vi "RPT_Convert Waveform.vi"(11 "Wave Data IN":dbl[][](array[numeric])) -> (0 "appended array":dbl[][](array[numeric]), 2 "Text OUT":string[][](array[string]), 3 "Count":i32)   [LabVIEW 2024]
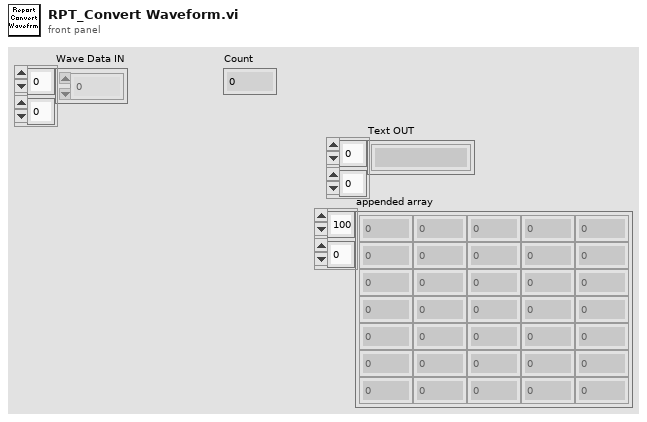
[diagram p1: front panel]
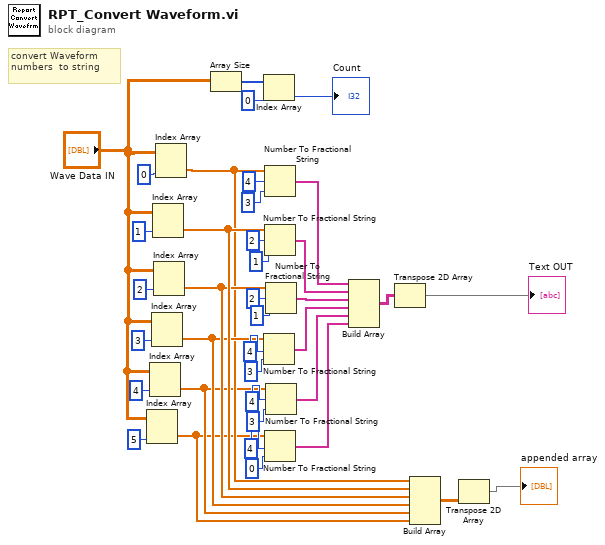
[diagram p0: block diagram]
diagram:
  # "convert Waveform\nnumbers  to string"
  n1 = Index Array(array="Wave Data IN", index (col)=5 ("index")) -> (element=w1:dbl[])  [unwired: 1 in]
  n2 = Index Array(array="Wave Data IN", index (col)=4 ("index")) -> (element=w2:dbl[])  [unwired: 1 in]
  n3 = Index Array(array="Wave Data IN", index (col)=3 ("index")) -> (element=w15:dbl[])  [unwired: 1 in]
  n4 = Index Array(array="Wave Data IN", index (col)=1 ("index")) -> (element=w17:dbl[])  [unwired: 1 in]
  n5 = Index Array(array="Wave Data IN", index (col)=2 ("index")) -> (element=w16:dbl[])  [unwired: 1 in]
  n6 = Index Array(array="Wave Data IN", index (col)=0 ("index")) -> (element=w12:dbl[])  [unwired: 1 in]
  n7 = Array Size(array="Wave Data IN") -> (size(s)=w26:i32[])
  n8 = Index Array(array=w26, index=0) -> (element=→"Count":i32)
  n9 = Number To Fractional String(number=w15, width (-)=i16 4 ("precision (6)"), precision (6)=i16 3) -> (F-format string=w36:string[])  [unwired: 1 in]
  n10 = Number To Fractional String(number=w12, width (-)=i16 4 ("precision (6)"), precision (6)=i16 3) -> (F-format string=w24:string[])  [unwired: 1 in]
  n11 = Number To Fractional String(number=w17, width (-)=i16 2 ("precision (6)"), precision (6)=i16 1) -> (F-format string=w30:string[])  [unwired: 1 in]
  n12 = Number To Fractional String(number=w1, width (-)=i16 4 ("precision (6)"), precision (6)=i16 0) -> (F-format string=w4:string[])  [unwired: 1 in]
  n13 = Number To Fractional String(number=w16, width (-)=i16 2 ("precision (6)"), precision (6)=i16 1) -> (F-format string=w35:string[])  [unwired: 1 in]
  n14 = Number To Fractional String(number=w2, width (-)=i16 4 ("precision (6)"), precision (6)=i16 3) -> (F-format string=w9:string[])  [unwired: 1 in]
  n15 = Build Array(w24, w30, w35, w36, w9, w4) -> (w37:string[][])
  n16 = Transpose 2D Array(2D array=w37) -> (transposed array=→"Text OUT":string[][])
  n17 = Build Array(w12, w17, w16, w15, w2, w1) -> (w19:dbl[][])
  n18 = Transpose 2D Array(2D array=w19) -> (transposed array=→"appended array":dbl[][])
